vi "Explain Query Plan.vi"(8 "error in (no error)":errorcluster, 11 "SQL Statement in":refnum<class "SQL Statement.lvclass">) -> (0 "error out":errorcluster, 2 "Query Plan":string, 3 "SQL Statement out":refnum<class "SQL Statement.lvclass">)   [LabVIEW 2011, in "SQLite.lvlib" / "SQL Statement.lvclass"]
uses:
  SQL Statement.lvclass
  SQL Connection/Connection.lvclass
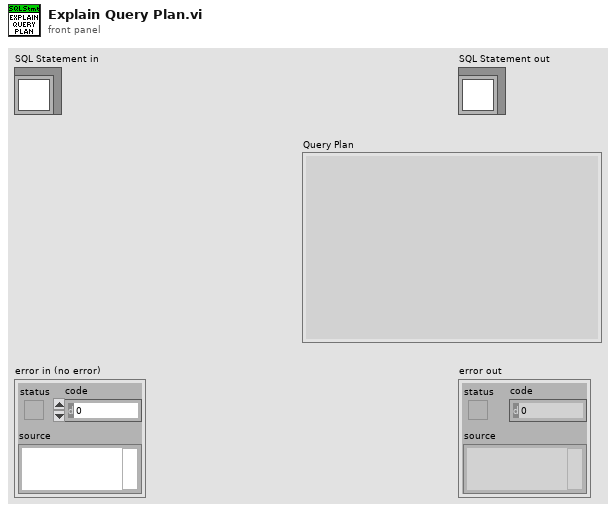
[diagram p1: front panel]
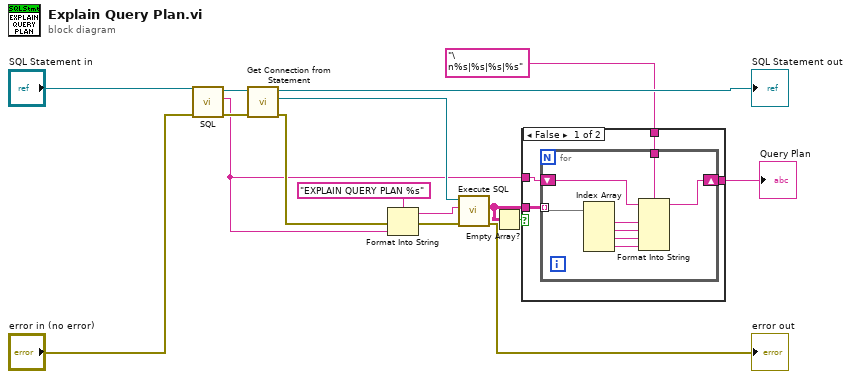
[diagram p0: block diagram]
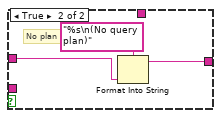
[diagram p2: hidden frame]
diagram:
  n1 = call "SQL.vi"("error in (no error)"="error in (no error)", "SQL Statement in"="SQL Statement in") -> ("error out"=w11:errorcluster, "SQL"=w3:string, "SQL Statement out"=w12:refnum<class "SQL Statement.lvclass">)  [unwired: 7 in]
  n2 = call "Get Connection from Statement.vi"("error in (no error)"=w11, "SQL Statement In"=w12) -> ("error out"=w6:errorcluster, "Connection out"=w9:refnum<class "Connection.lvclass">, "SQL Statement Out"=→"SQL Statement out":refnum<class "SQL Statement.lvclass">)  [unwired: 7 in]
  n3 = Format Into String(format string="EXPLAIN QUERY PLAN %s", error in=w6, w3) -> (resulting string=w8:string, error out=w7:errorcluster)  [unwired: 1 in]
  n4 = call "Execute SQL.vi"("error in (no error)"=w7, "SQL"=w8, "SQLite Connection in"=w9) -> ("error out"=→"error out":errorcluster, "Result Set"=w2:string[][])  [unwired: 5 in, 2 out]
  n5 = Empty Array?(array=w2) -> (empty?=w1:bool)
  n6 = case shown="False" w1 {
    tunnel: w2 -> [w20 _]
    tunnel: "\n%s|%s|%s|%s" ("format string") -> [w19 _]
    tunnel: [w18 w31] -> w4
    tunnel: w3 -> [w17 w30]
    frame False {
      n7 = for {
        tunnel: w20 -> [w28] mode=indexing
        tunnel: w19 -> [w23]
        shift-right: [w22] -> w18
        shift-left: w17 -> [w21]
        n8 = Index Array(array=w28) -> (element #1=w27:string, element #2=w26:string, element #3=w25:string, element #4=w24:string)  [unwired: 4 in]
        n9 = Format Into String(format string=w23, initial string=w21, w27, w26, w25, w24) -> (resulting string=w22:string)  [unwired: 1 in, 1 out]
      }
    }
    frame True {
      # "No plan"
      n10 = Format Into String(format string="%s\n(No query plan)", w30) -> (resulting string=w31:string)  [unwired: 2 in, 1 out]
    }
  }
  "Query Plan" <- w4
